vi "Unitherm_Test Process.vi"() -> ()   [LabVIEW 2015]
panel:
  in  "error in":errorcluster
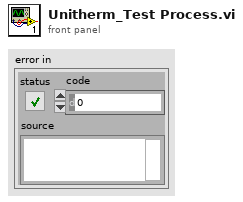
[diagram p1: front panel]
types:
  T1 = typedef "Control_General Command Cluster.ctl" = cluster{"Caller-Q":refnum<queue>, "Command":string, "Return":string, "Data":variant, "Timeout":dbl}
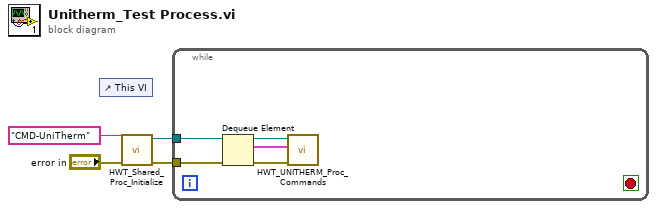
[diagram p0: block diagram]
diagram:
  n1 = control-ref of="This VI"() -> ()  [unwired: 1 out]
  n2 = call "HWT_Shared_Proc_Initialize.vi"("error in (no error)"="error in", "Q-Name"="CMD-UniTherm") -> ("error out"=w1:errorcluster, "Queue out"=w2:refnum<queue>)  [unwired: 8 in]
  n3 = while {
    tunnel: w2 -> [w9]
    tunnel: w1 -> [w8]
    stop <- _ stop-if-true
    n4 = Dequeue Element(queue=w9, error in (no error)=w8) -> (queue out=w7:refnum<queue>, element=w6:T1, error out=w5:errorcluster)  [unwired: 1 in, 1 out]
    n5 = call "HWT_UNITHERM_Proc_Commands.vi"("error in (no error)"=w5, "Settings"=w6, "Queue in"=w7) -> ()  [unwired: 8 in, 1 out]
  }
